vi "Position Feedback.vi"() -> ()   [LabVIEW 2020]
uses:
  Classes/Controller/Controller.lvclass
  Classes/Controller/Motion/A3200/A3200.lvclass
panel:
  in  "stop":bool
  out "XYZTheta Out":dbl[](array[numeric])
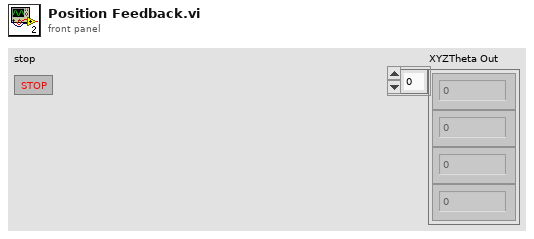
[diagram p1: front panel]
types:
  T1 = typedef "Controller.lvclass/Controllers.ctl" = cluster{"I-O.lvclass":refnum<class "I-O.lvclass">, "Gantry":refnum<k24>, "Dispenser":refnum<visa-resource-name>}
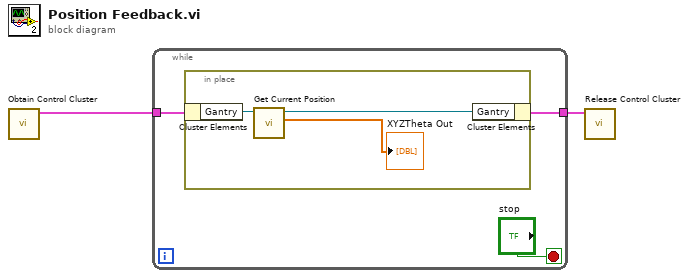
[diagram p0: block diagram]
diagram:
  n1 = call "Obtain Control Cluster.vi"() -> ("Control Out"=w2:T1)  [unwired: 11 in]
  n2 = while {
    tunnel: w2 -> [w5]
    tunnel: [w4] -> w1
    stop <- "stop" stop-if-true
    n3 = in-place {
      n4 = in-place-cluster #1(w5) -> ("Gantry"=w8:refnum<k24>)
      n5 = call "Get Current Position.vi"("Gantry In"=w8) -> ("XYZTheta Out"=→"XYZTheta Out":dbl[], "Gantry Out"=w7:refnum<k24>)  [unwired: 8 in, 1 out]
      n6 = in-place-cluster #1("Gantry"=w7) -> (w4:T1)
    }
  }
  n7 = call "Release Control Cluster.vi"("output cluster"=w1) -> ()  [unwired: 11 in]
